vi "Analyzer.GetWord_FGV.vi"(7 "Operation":enum16{"Reset", "Get"}(ring), 10 "List of Words":string[](array[string])) -> (2 "Word for search":string)   [LabVIEW 2022 SP3, in "Analyzer.lvclass"]
uses:
  Analyzer.lvclass
  Analyzer.lvclass/Analyzer.ctl
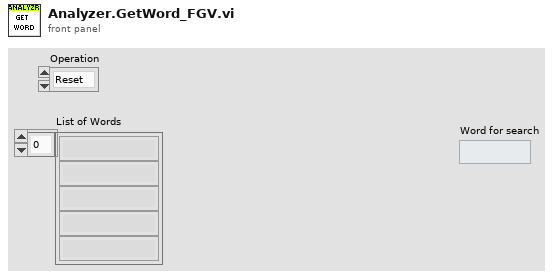
[diagram p1: front panel]
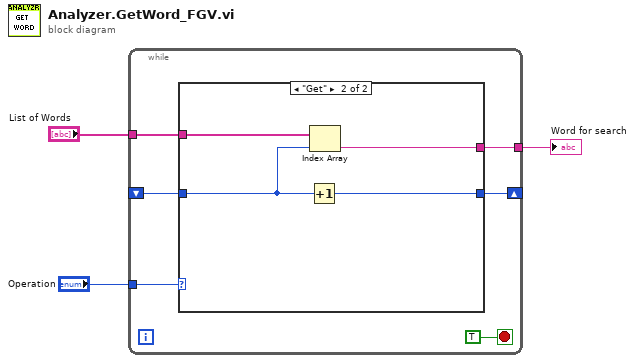
[diagram p0: block diagram]
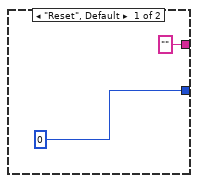
[diagram p2: hidden frame]
diagram:
  n1 = while {
    tunnel: "Operation" -> [w9]
    shift-right: [w8] -> _
    shift-left: _ -> [w5]
    tunnel: "List of Words" -> [w7]
    tunnel: [w4] -> w1
    stop <- TRUE stop-if-true
    n2 = case shown="\"Get\"" w9 {
      tunnel: [0 w13] -> w8
      tunnel: w7 -> [_ w15]
      tunnel: w5 -> [_ w14]
      tunnel: ["" ("String") w12] -> w4
      frame "Reset", Default {
      }
      frame "Get" {
        n3 = Increment(x=w14) -> (x+1=w13:i32)
        n4 = Index Array(array=w15, index=w14) -> (element=w12:string)
      }
    }
  }
  "Word for search" <- w1
